vi "ABR-Update Run Number.vi"(8 "Resume":bool, 10 "CAP or ABR":enum16{"CAP", "ABR"}(ring)=enum."ABR" caption="Measure what", 11 "State (in)":T1) -> (0 "raw data filestem":path, 2 "run #":i16, 3 "State (out)":T1)   [LabVIEW 2020]
uses:
  CFTS SubVIs/CFTS-Experiment State.ctl
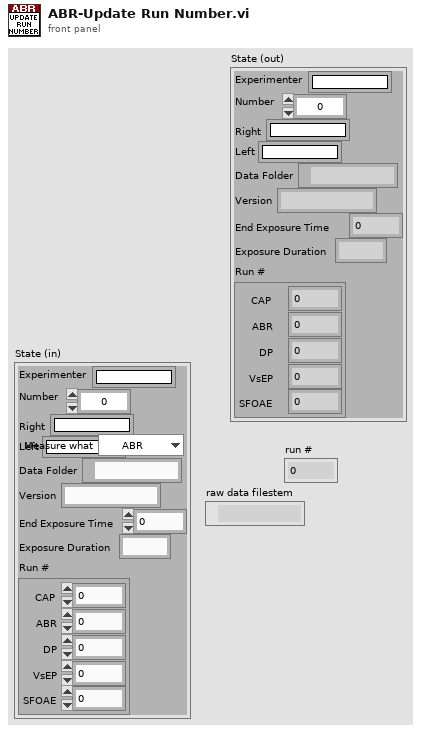
[diagram p1: front panel]
types:
  T1 = typedef "CFTS-Experiment State.ctl" = cluster{"Experimenter":string, "Number":u32, "Right":string, "Left":string, "Data Folder":path, "Version":string, "End Exposure Time":dbl, "Exposure Duration":string, "Run #":cluster{"CAP":i32, "ABR":i32, "DP":i32, "VsEP":i32, "SFOAE":i32}}
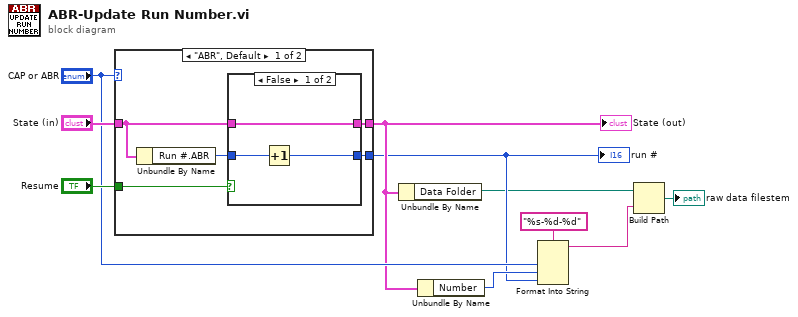
[diagram p0: block diagram]
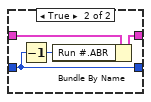
[diagram p2: hidden frame]
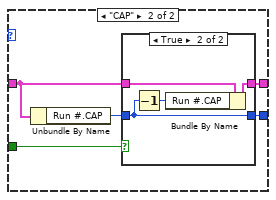
[diagram p3: hidden frame]
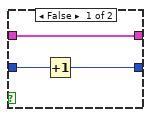
[diagram p4: hidden frame]
diagram:
  n1 = case shown="\"ABR\", Default" "CAP or ABR" {
    tunnel: "State (in)" -> [w12 w24]
    tunnel: "Resume" -> [w15 w27]
    tunnel: [w13 w25] -> w4
    tunnel: [w11 w23] -> w6
    frame "ABR", Default {
      n2 = Unbundle By Name(w12) -> ("Run #.ABR"=w14:i32)
      n3 = case shown="False" w15 {
        tunnel: w14 -> [w18 w21]
        tunnel: [w17 w21] -> w13
        tunnel: w12 -> [w16 w22]
        tunnel: [w16 w19] -> w11
        frame False {
          n4 = Increment(x=w18) -> (x+1=w17:i32)
        }
        frame True {
          n5 = Decrement(x=w21) -> (x-1=w20:i32)
          n6 = Bundle By Name(cluster=w22, "Run #.ABR"=w20) -> (w19:T1)
        }
      }
    }
    frame "CAP" {
      n7 = Unbundle By Name(w24) -> ("Run #.CAP"=w26:i32)
      n8 = case shown="True" w27 {
        tunnel: w26 -> [w30 w33]
        tunnel: [w29 w33] -> w25
        tunnel: w24 -> [w28 w34]
        tunnel: [w28 w31] -> w23
        frame False {
          n9 = Increment(x=w30) -> (x+1=w29:i32)
        }
        frame True {
          n10 = Decrement(x=w33) -> (x-1=w32:i32)
          n11 = Bundle By Name(cluster=w34, "Run #.CAP"=w32) -> (w31:T1)
        }
      }
    }
  }
  "run #" <- w4
  "State (out)" <- w6
  n12 = Unbundle By Name(w6) -> ("Data Folder"=w3:path)
  n13 = Unbundle By Name(w6) -> ("Number"=w5:u32)
  n14 = Format Into String(format string="%s-%d-%d", "CAP or ABR", w5, w4) -> (resulting string=w2:string)  [unwired: 2 in, 1 out]
  n15 = Build Path(base path=w3, name or relative path=w2) -> (appended path=→"raw data filestem":path)
